vi "SnoUserLineNumber.vi"(1 "Numeric":i32) -> (0 "line":T1)   [LabVIEW 2013]
uses:
  <vilib>/Rock Robotics/WPI/DriverStation/DriverStationLCD/WPI_DriverStationLCDLCDLine.ctl
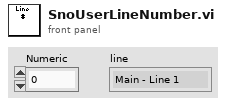
[diagram p1: front panel]
types:
  T1 = typedef "WPI_DriverStationLCDLCDLine.ctl" = enum16{"Main - Line 1", "User - Line 2", "User - Line 3", "User - Line 4", "User - Line 5", "User - Line 6"}
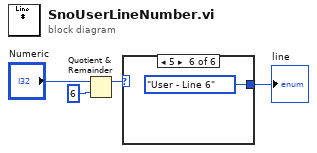
[diagram p0: block diagram]
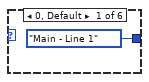
[diagram p2: hidden frame]
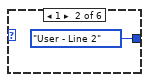
[diagram p3: hidden frame]
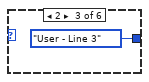
[diagram p4: hidden frame]
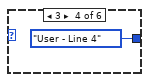
[diagram p5: hidden frame]
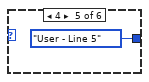
[diagram p6: hidden frame]
diagram:
  n1 = Quotient & Remainder(x="Numeric", y=6) -> (x-y*floor(x/y)=w3:i32)  [unwired: 1 out]
  n2 = case shown="5" w3 {
    tunnel: [WPI_DriverStationLCDLCDLine."Main - Line 1" ("line") WPI_DriverStationLCDLCDLine."User - Line 2" ("line") WPI_DriverStationLCDLCDLine."User - Line 3" ("line") WPI_DriverStationLCDLCDLine."User - Line 4" ("line") WPI_DriverStationLCDLCDLine."User - Line 5" ("line") WPI_DriverStationLCDLCDLine."User - Line 6" ("line")] -> w4
    frame 0, Default {
    }
    frame 1 {
    }
    frame 2 {
    }
    frame 3 {
    }
    frame 4 {
    }
    frame 5 {
    }
  }
  "line" <- w4
